vi "menu-InterleaveSeperators.vi"(11 "Array":cluster{"element":T1[]}[](array[cluster])) -> (3 "element":T1[](array[typedef]))   [LabVIEW 2019]
uses:
  <resource>/Framework/Providers/API/mxLvMenuItem.ctl
  5d9bda2c-eec2-4e57-8110-4fc90c1cf2bd.vi
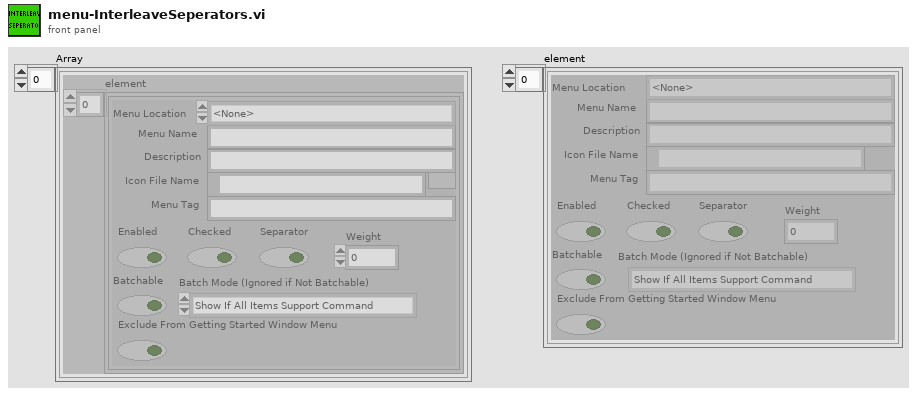
[diagram p1: front panel]
types:
  T1 = typedef "mxLvMenuItem.ctl" = cluster{"Menu Name":string, "Description":string, "Icon File Name":path, "Menu Tag":string, "Enabled":bool, "Checked":bool, "Separator":bool, "Batchable":bool, "Weight":i32, "Batch Mode (Ignored if Not Batchable)":enum32{"Show If All Items Support Command", "Show If Any Items Support Command"}, "Menu Location":enum32{"<None>", "Project", "Project / Build Specifications", "Tools", "Tools / Source Control", "Tools / Real-Time Module", "Help"}, "Exclude From Getting Started Window Menu":bool}
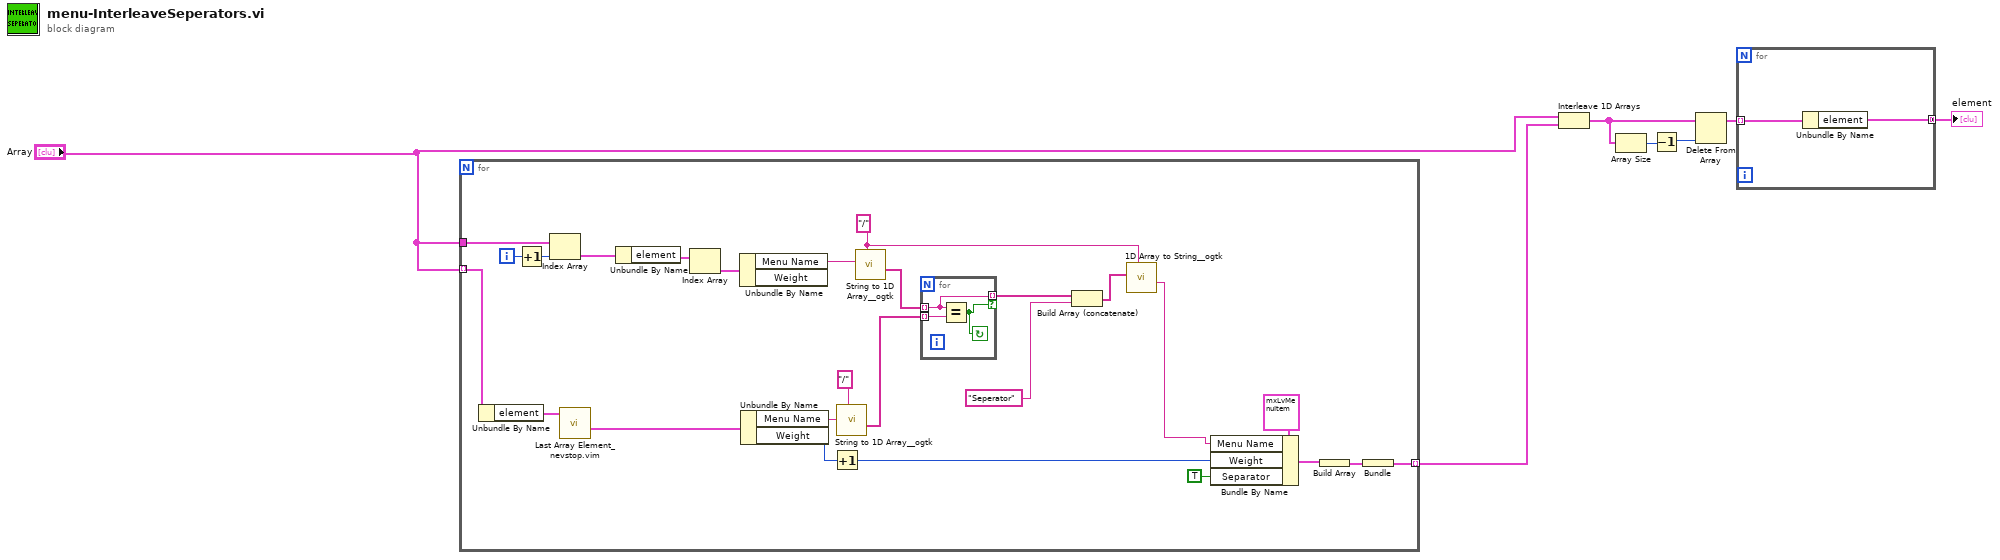
[diagram p0: block diagram]
diagram:
  n1 = for {
    tunnel: "Array" -> [w33] mode=indexing
    tunnel: [w23] -> w5 mode=indexing
    tunnel: "Array" -> [w22]
    i -> [w21]
    w15 = "/" ("delimiter (Tab)")
    n2 = Unbundle By Name(w33) -> ("element"=w32:T1[])
    n3 = Increment(x=w21) -> (x+1=w20:i32)
    n4 = Index Array(array=w22, index=w20) -> (element=w19:cluster{"element":T1[]})
    n5 = call "Last Array Element_nevstop.vim"("Array"=w32) -> ("Last Element"=w17:T1)  [unwired: 10 in]
    n6 = Unbundle By Name(w19) -> ("element"=w18:T1[])
    n7 = Index Array(array=w18) -> (element=w16:T1)  [unwired: 1 in]
    n8 = Unbundle By Name(w16) -> ("Menu Name"=w14:string)  [unwired: 1 out]
    n9 = Unbundle By Name(w17) -> ("Menu Name"=w28:string, "Weight"=w30:i32)
    n10 = Increment(x=w30) -> (x+1=w29:i32)
    n11 = call <userlib>:"String to 1D Array__ogtk.vi"("delimiter (Tab)"="/", "string"=w28) -> ("Array of Strings"=w12:string[])  [unwired: 9 in]
    n12 = call <userlib>:"String to 1D Array__ogtk.vi"("delimiter (Tab)"=w15, "string"=w14) -> ("Array of Strings"=w13:string[])  [unwired: 9 in]
    n13 = for {
      tunnel: w13 -> [w35] mode=indexing
      tunnel: w12 -> [w36] mode=indexing
      tunnel: [w35] -> w11 mode=indexing if=w34
      stop <- w34 continue-if-true
      n14 = Equal?(x=w35, y=w36) -> (x = y?=w34:bool)
    }
    n15 = Build Array (concatenate)(w11, "Seperator" ("delimiter (Tab)")) -> (w10:string[])
    n16 = call <userlib>:"1D Array to String__ogtk.vi"("delimiter (Tab)"=w15, "Array of Strings"=w10) -> ("delimited string"=w9:string)  [unwired: 9 in]
    n17 = Bundle By Name(cluster=T1 {"Menu Name"="Seperator", "Description"="", "Icon File Name"=path "", "Menu Tag"="", "Enabled"=TRUE, "Checked"=FALSE, "Separator"=TRUE, "Batchable"=FALSE, "Weight"=0, "Batch Mode (Ignored if Not Batchable)"=enum."Show If All Items Support Command", "Menu Location"=enum."<None>", "Exclude From Getting Started Window Menu"=FALSE} ("Menu Item"), "Menu Name"=w9, "Weight"=w29, "Separator"=TRUE) -> (w25:T1)
    n18 = Build Array(w25) -> (w24:T1[])
    n19 = Bundle(w24) -> (w23:cluster{T1[]})  [unwired: 1 in]
  }
  n20 = Interleave 1D Arrays("Array", w5) -> (w2:cluster{"element":T1[]}[])
  n21 = Array Size(array=w2) -> (size(s)=w4:i32)
  n22 = Decrement(x=w4) -> (x-1=w3:i32)
  n23 = Delete From Array(array=w2, index=w3) -> (array with subset deleted=w6:cluster{"element":T1[]}[])  [unwired: 1 in, 1 out]
  n24 = for {
    tunnel: w6 -> [w38] mode=indexing
    tunnel: [w37] -> w7 mode=concatenating
    n25 = Unbundle By Name(w38) -> ("element"=w37:T1[])
  }
  "element" <- w7
